vi "my.vi"() -> ()   [LabVIEW 2015]
uses:
  <vilib>/NXT/Block Support/NXT_InputPort.ctl
  <vilib>/NXT/Block Support/NXT_OutputPort.ctl
  <vilib>/NXT/Dual Mode Library/Sensors/Sonar_cm.vi
  <vilib>/NXT/Dual Mode Library/Sensors/Light_On.vi
  <vilib>/NXT/NXTIO Xnodes/NXTIONodeSubVIs/NXTMoveMotors.vi
  <vilib>/NXT/Dual Mode Library/Waits/Wait_Num.vi
  <vilib>/NXT/NXTIO Xnodes/AddressXNode/NXTIOAddress.xnode
  <vilib>/NXT/Subs/LVHSConnector.ctl
  <vilib>/NXT/NXTIO Xnodes/NXTIOXNode/NXTIO.xnode
  <vilib>/NXT/LegoClasses/BrickReference/BrickReference.lvclass
panel:
  in  "stop":bool
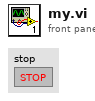
[diagram p1: front panel]
types:
  T1 = typedef "NXT_InputPort.ctl" = u32
  T2 = typedef "NXT_OutputPort.ctl" = u8
  T3 = typedef "LVHSConnector.ctl" = refnum<class "BrickReference.lvclass">
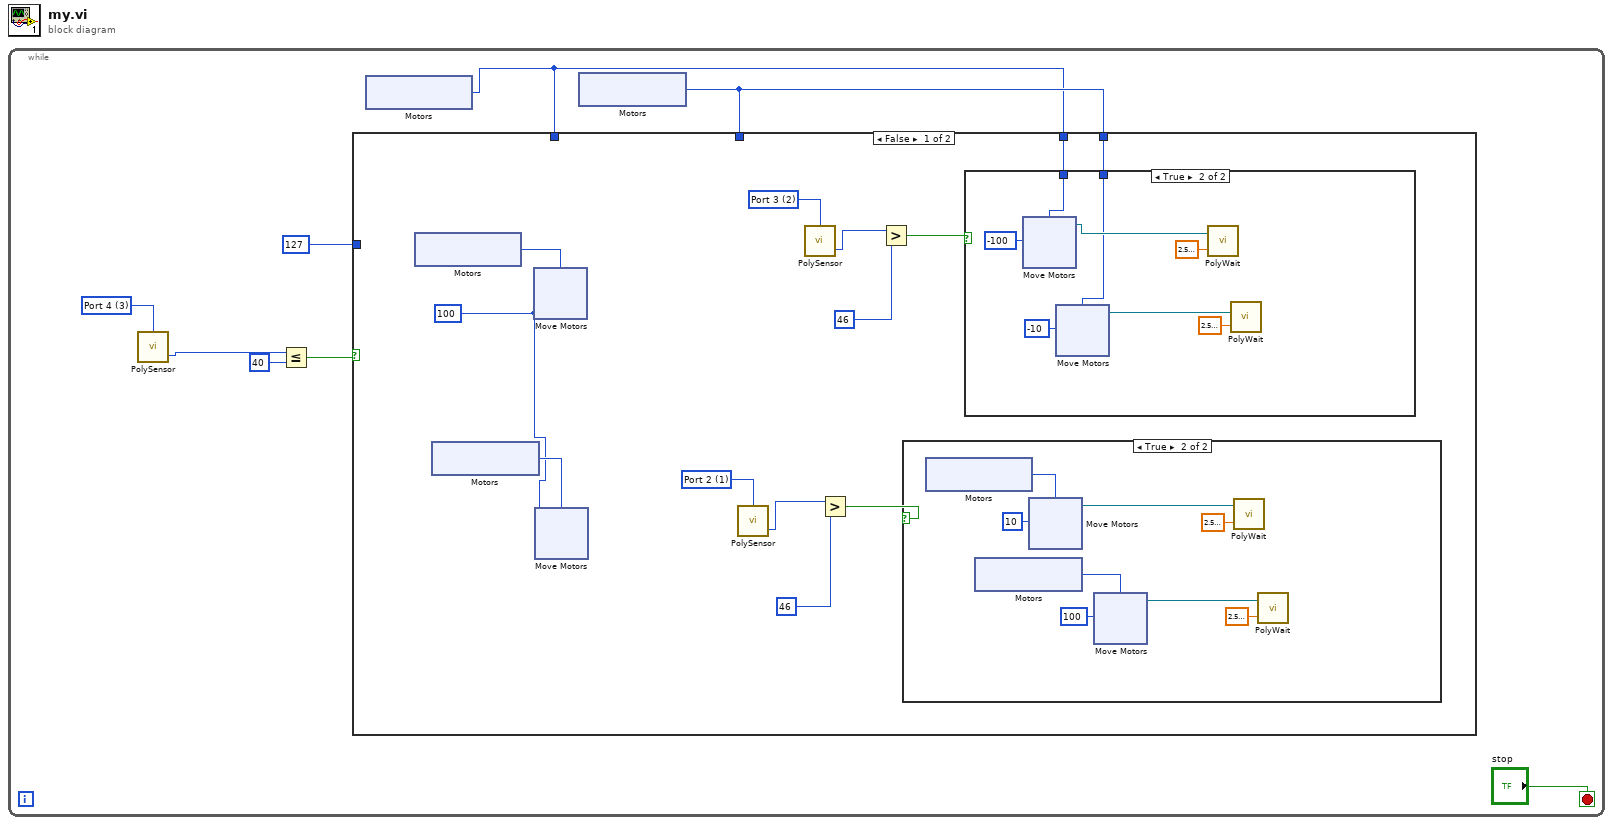
[diagram p0: block diagram]
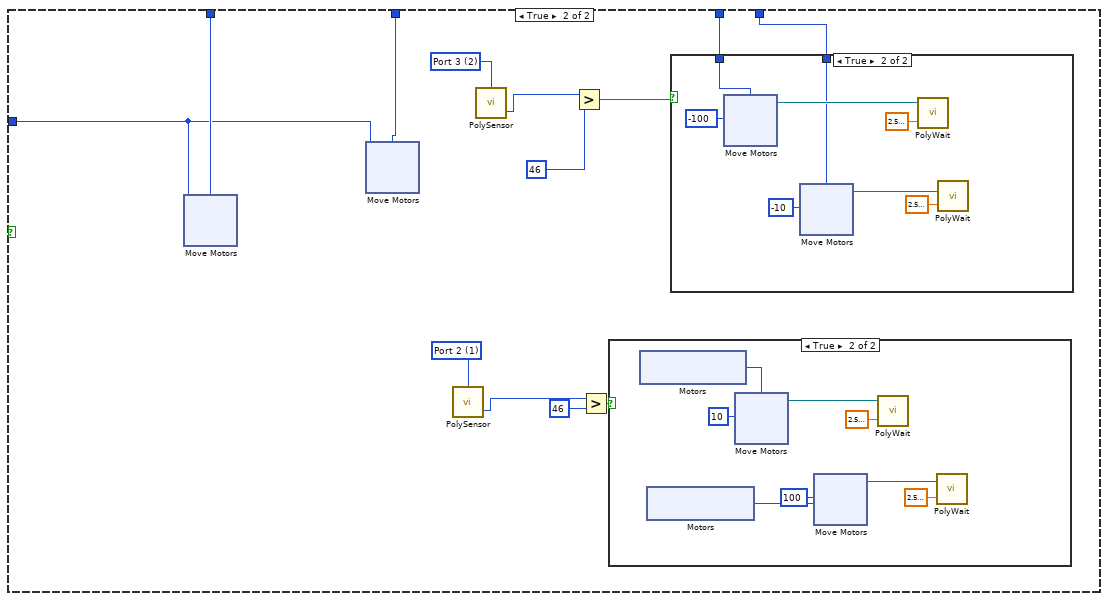
[diagram p4: hidden frame]
diagram:
  n1 = while {
    stop <- "stop" stop-if-true
    w8 = T1 3 items=["Port 1", "Port 2", "Port 3", "Port 4"] ("Port (Port 4)")
    n2 = call-poly <vilib>:"PolySensor.vi"("Port (Port 4)"=w8) -> ("Distance (cm)"=w7:i16)  [unwired: 2 in, 1 out]
    n3 = Less Or Equal?(x=w7, y=i16 40) -> (x <= y?=w5:bool)
    n4 = xnode "Motors"() -> ("Motor"=w2:T2)
    n5 = xnode "Motors"() -> ("Motor"=w3:T2)
    n6 = case shown="False" w5 {
      tunnel: w2 -> [_ w98]
      tunnel: w3 -> [_ w97]
      tunnel: i8 127 ("Power/Speed 1") -> [_ w96]
      tunnel: w3 -> [w11 w90]
      tunnel: w2 -> [w12 w91]
      frame False {
        w13 = T1 1 items=["Port 1", "Port 2", "Port 3", "Port 4"] ("Port (Port 3)")
        w20 = T1 2 items=["Port 1", "Port 2", "Port 3", "Port 4"] ("Port (Port 3)")
        w21 = i8 100 ("Power/Speed 1")
        n7 = xnode "Motors"() -> ("Motor"=w23:T2)
        n8 = xnode "Motors"() -> ("Motor"=w22:T2)
        n9 = xnode "Move Motors"("Power/Speed 1"=w21, "Motors"=w23) -> ()  [unwired: 1 in, 1 out]
        n10 = xnode "Move Motors"("Power/Speed 1"=w21, "Motors"=w22) -> ()  [unwired: 1 in, 1 out]
        n11 = call-poly <vilib>:"PolySensor.vi"("Port (Port 3)"=w13) -> ("Scaled Value"=w15:i16)  [unwired: 2 in, 1 out]
        n12 = call-poly <vilib>:"PolySensor.vi"("Port (Port 3)"=w20) -> ("Scaled Value"=w18:i16)  [unwired: 2 in, 1 out]
        n13 = Greater?(x=w15, y=i16 46) -> (0:w16:bool)
        n14 = Greater?(x=w18, y=i16 46) -> (0:w19:bool)
        n15 = case shown="True" w16 {
          frame False {
          }
          frame True {
            n16 = xnode "Motors"() -> ("Motor"=w29:T2)
            n17 = xnode "Motors"() -> ("Motor"=w28:T2)
            n18 = xnode "Move Motors"("Power/Speed 1"=i8 10, "Motors"=w29) -> ("NXT/EV3"=w31:T3)  [unwired: 1 in]
            n19 = xnode "Move Motors"("Power/Speed 1"=i8 100, "Motors"=w28) -> ("NXT/EV3"=w30:T3)  [unwired: 1 in]
            n20 = call-poly <vilib>:"PolyWait.vi"("Time (1 sec)"=sgl 2.6, "NXT/EV3"=w31) -> ()  [unwired: 2 in, 1 out]
            n21 = call-poly <vilib>:"PolyWait.vi"("Time (1 sec)"=sgl 2.6, "NXT/EV3"=w30) -> ()  [unwired: 2 in, 1 out]
          }
        }
        n22 = case shown="True" w19 {
          tunnel: w12 -> [_ w53]
          tunnel: w11 -> [_ w52]
          frame False {
          }
          frame True {
            n23 = xnode "Move Motors"("Power/Speed 1"=i8 -100, "Motors"=w53) -> ("NXT/EV3"=w55:T3)  [unwired: 1 in]
            n24 = xnode "Move Motors"("Power/Speed 1"=i8 -10, "Motors"=w52) -> ("NXT/EV3"=w54:T3)  [unwired: 1 in]
            n25 = call-poly <vilib>:"PolyWait.vi"("Time (1 sec)"=sgl 2.6, "NXT/EV3"=w55) -> ()  [unwired: 2 in, 1 out]
            n26 = call-poly <vilib>:"PolyWait.vi"("Time (1 sec)"=sgl 2.6, "NXT/EV3"=w54) -> ()  [unwired: 2 in, 1 out]
          }
        }
      }
      frame True {
        w89 = T1 1 items=["Port 1", "Port 2", "Port 3", "Port 4"] ("Port (Port 3)")
        w92 = T1 2 items=["Port 1", "Port 2", "Port 3", "Port 4"] ("Port (Port 3)")
        n27 = xnode "Move Motors"("Power/Speed 1"=w96, "Motors"=w98) -> ()  [unwired: 1 in, 1 out]
        n28 = xnode "Move Motors"("Power/Speed 1"=w96, "Motors"=w97) -> ()  [unwired: 1 in, 1 out]
        n29 = call-poly <vilib>:"PolySensor.vi"("Port (Port 3)"=w89) -> ("Scaled Value"=w87:i16)  [unwired: 2 in, 1 out]
        n30 = call-poly <vilib>:"PolySensor.vi"("Port (Port 3)"=w92) -> ("Scaled Value"=w95:i16)  [unwired: 2 in, 1 out]
        n31 = Greater?(x=w95, y=i16 46) -> (0:w93:bool)
        n32 = Greater?(x=w87, y=i16 46) -> (0:w88:bool)
        n33 = case shown="True" w88 {
          frame False {
          }
          frame True {
            n34 = xnode "Motors"() -> ("Motor"=w106:T2)
            n35 = xnode "Motors"() -> ("Motor"=w105:T2)
            n36 = xnode "Move Motors"("Power/Speed 1"=i8 10, "Motors"=w106) -> ("NXT/EV3"=w104:T3)  [unwired: 1 in]
            n37 = xnode "Move Motors"("Power/Speed 1"=i8 100, "Motors"=w105) -> ("NXT/EV3"=w103:T3)  [unwired: 1 in]
            n38 = call-poly <vilib>:"PolyWait.vi"("Time (1 sec)"=sgl 2.6, "NXT/EV3"=w104) -> ()  [unwired: 2 in, 1 out]
            n39 = call-poly <vilib>:"PolyWait.vi"("Time (1 sec)"=sgl 2.6, "NXT/EV3"=w103) -> ()  [unwired: 2 in, 1 out]
          }
        }
        n40 = case shown="True" w93 {
          tunnel: w91 -> [_ w128]
          tunnel: w90 -> [_ w127]
          frame False {
          }
          frame True {
            n41 = xnode "Move Motors"("Power/Speed 1"=i8 -100, "Motors"=w128) -> ("NXT/EV3"=w129:T3)  [unwired: 1 in]
            n42 = xnode "Move Motors"("Power/Speed 1"=i8 -10, "Motors"=w127) -> ("NXT/EV3"=w130:T3)  [unwired: 1 in]
            n43 = call-poly <vilib>:"PolyWait.vi"("Time (1 sec)"=sgl 2.6, "NXT/EV3"=w129) -> ()  [unwired: 2 in, 1 out]
            n44 = call-poly <vilib>:"PolyWait.vi"("Time (1 sec)"=sgl 2.6, "NXT/EV3"=w130) -> ()  [unwired: 2 in, 1 out]
          }
        }
      }
    }
  }
